vi "Write Command Processor Status.vi"(8 "error in (no error)":errorcluster, 10 "Command Processor Status":T1, 11 "Command Processor in":refnum<class "Command Processor.lvclass">) -> (0 "error out":errorcluster, 3 "Command Processor out":refnum<class "Command Processor.lvclass">)   [LabVIEW 2013, in "Command Processor.lvlib" / "Command Processor.lvclass"]
uses:
  Command Processor.lvclass
  Command Processor Status.ctl
  Current Previous State Status.ctl
  State Status.ctl
  Command/Command Status.ctl
  Command/State Status.ctl
  <vilib>/ActorFramework/Actor/Actor.lvclass/Actor.ctl
  Command Processor.lvclass/Command Processor.ctl
  System Messages/New Command Processor Status Msg/New Command Processor Status Msg.lvclass/New Command Processor Status Msg.ctl
  <vilib>/ActorFramework/Message Enqueuer/Message Enqueuer.lvclass/Message Enqueuer.ctl
  <vilib>/ActorFramework/Message Enqueuer/Enqueue.vi
  <vilib>/ActorFramework/Message Priority Queue/Priority Enqueue.vi
  System Messages/New Command Processor Status Msg/New Command Processor Status Msg.lvclass
  <vilib>/ActorFramework/Actor/Actor.lvclass
  Command/Command.lvclass
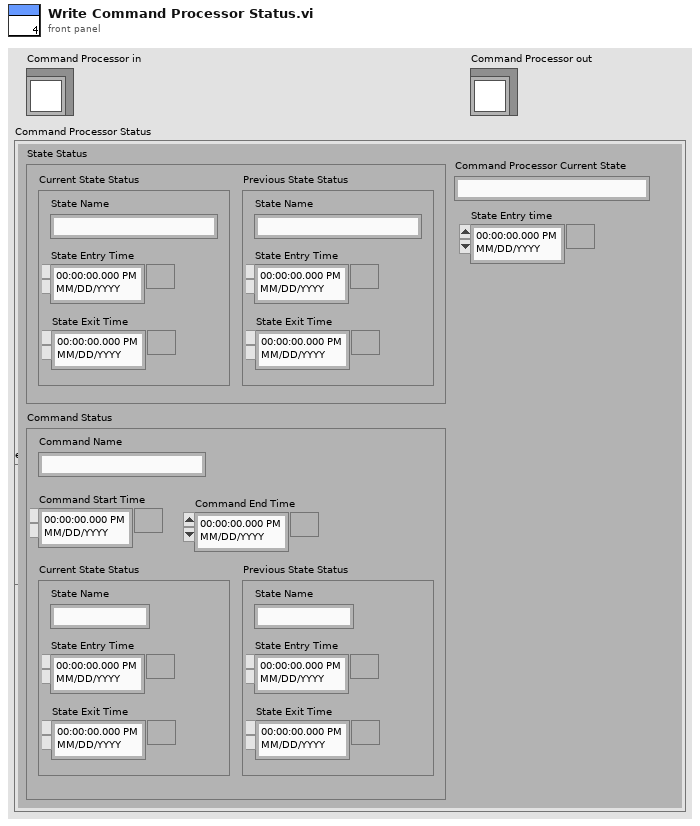
[diagram p1: front panel]
types:
  T1 = typedef "Command Processor.lvlib/Command Processor.lvclass/Command Processor Status.ctl" = cluster{"State Entry time":timestamp, "State Status":T2, "Command Processor Current State":string, "Command Status":T4}
  T2 = typedef "Current Previous State Status.ctl" = cluster{"Current State Status":T3, "Previous State Status":T3}
  T3 = typedef "State Status.ctl" = cluster{"State Name":string, "State Entry Time":timestamp, "State Exit Time":timestamp}
  T4 = typedef "Command Processor.lvlib/Command.lvlib/Command.lvclass/Command Status.ctl" = cluster{"Command Name":string, "Current State Status":T5, "Command Start Time":timestamp, "Command End Time":timestamp, "Previous State Status":T5}
  T5 = typedef "Command Processor.lvlib/Command.lvlib/Command.lvclass/State Status.ctl" = cluster{"State Name":string, "State Entry Time":timestamp, "State Exit Time":timestamp}
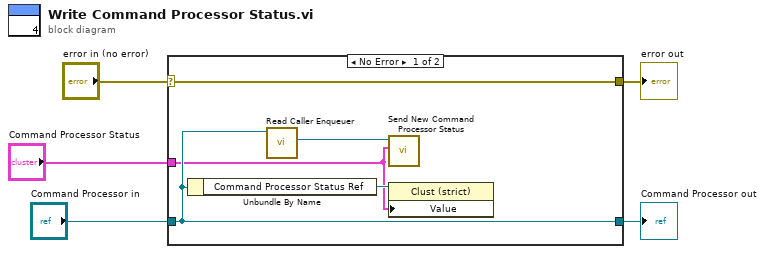
[diagram p0: block diagram]
diagram:
  n1 = case shown="No Error" "error in (no error)" {
    selector: "error in (no error)" -> [w10 w12]
    tunnel: [w10 w12] -> w4
    tunnel: [w8 w11] -> w2
    tunnel: "Command Processor in" -> [w8 w11]
    tunnel: "Command Processor Status" -> [w6 _]
    frame No Error {
      n2 = Unbundle By Name(w8) -> ("Command Processor Status Ref"=w9:refnum<vi>)
      n3 = call <vilib>:"Read Caller Enqueuer.vi"("Actor"=w8) -> ("Caller Enqueuer"=w7:refnum<class "Message Enqueuer.lvclass">)  [unwired: 10 in]
      n4 = call "Send New Command Processor Status.vi"("Command Processor Status"=w6, "Message Enqueuer"=w7) -> ()  [unwired: 8 in, 2 out]
      n5 = property class="Clust (strict)"(reference=w9, "Value"=w6) -> ()  [unwired: 1 in, 2 out]
    }
    frame Error {
    }
  }
  "error out" <- w4
  "Command Processor out" <- w2
